vi "Fetch Measurement.vi"(8 "error in (no error)":errorcluster, 11 "VISA resource name":refnum<visa-resource-name>) -> (0 "error out":errorcluster, 2 "Measured Value":dbl, 3 "VISA resource name out":refnum<visa-resource-name>)   [LabVIEW 2013, in "DmmPwr Simulator.lvlib"]
doc: "Fetches the measurement.\n\n<B>Note:</B>\nThis VI does not check the instrument status. Typically, you call this VI only in a sequence of calls to other low-level instrument driver VIs. The sequence performs one operation. You use the low-level VIs to optimize one or more aspects of interaction with the instrument. If you want to check the instrument status, call the <B>Error Query VI</B> at the conclusion of the sequence."
uses:
  <instrlib>/DmmPwr Simulator/DmmPwr Simulator.lvlib
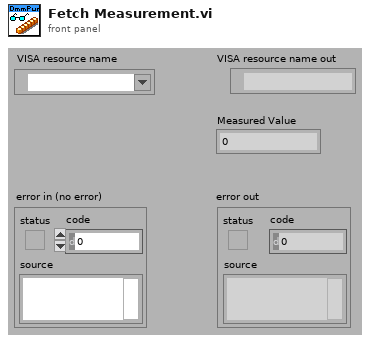
[diagram p1: front panel]
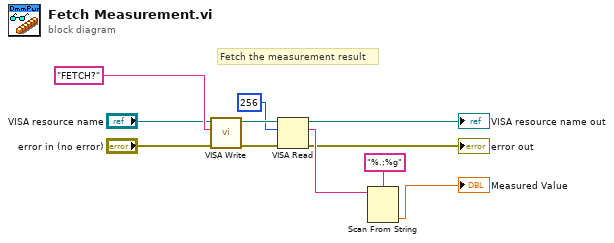
[diagram p0: block diagram]
diagram:
  # "Fetch the measurement result"
  n1 = call <instrlib>:"VISA Write.vi"("error in"="error in (no error)", "write buffer"="FETCH?", "VISA resource name"="VISA resource name") -> ("error out"=w7:errorcluster, "VISA resource name out"=w8:refnum<visa-resource-name>)  [unwired: 6 in, 1 out]
  n2 = VISA Read(VISA resource name=w8, byte count=u32 256, error in (no error)=w7) -> (VISA resource name out=→"VISA resource name out":refnum<visa-resource-name>, read buffer=w5:string, error out=→"error out":errorcluster)  [unwired: 1 out]
  n3 = Scan From String(format string="%.;%g", input string=w5) -> (output 1=→"Measured Value":dbl)  [unwired: 2 in, 4 out]
